vi "Delete Channel Refnum.vi"(8 "error in (no error)":errorcluster, 11 "Channel":T1) -> (0 "error out":errorcluster, 3 "LIBSSH2_CHANNEL*":u64)   [LabVIEW 2013, in "libssh2.lvlib"]
uses:
  libssh2.lvlib
  Channel Refnum.ctl
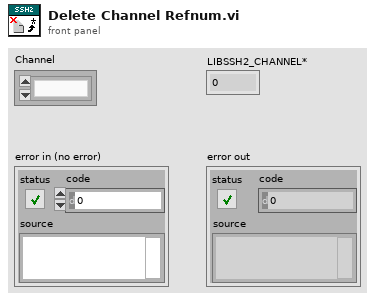
[diagram p1: front panel]
types:
  T1 = typedef "libssh2.lvlib/Channel Refnum.ctl" = refnum<k1>
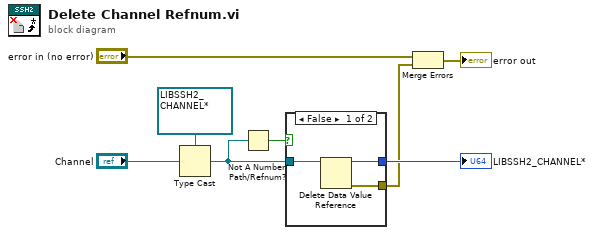
[diagram p0: block diagram]
diagram:
  n1 = Type Cast(type=refnum<data-value> refnum ("data value reference"), x="Channel") -> (*(type *) &x=w4:refnum<data-value>)
  n2 = Not A Number/Path/Refnum?(number/path/refnum=w4) -> (NaN/Path/Refnum?=w3:bool)
  n3 = case shown="False" w3 {
    tunnel: [w11 _] -> w6
    tunnel: [w10 _] -> w5
    tunnel: w4 -> [w9 _]
    frame False {
      n4 = Delete Data Value Reference(data value reference=w9) -> (data value=w11:u64, error out=w10:errorcluster)  [unwired: 1 in]
    }
    frame True {
    }
  }
  "LIBSSH2_CHANNEL*" <- w6
  n5 = Merge Errors("error in (no error)", w5) -> (→"error out":errorcluster)
